vi "Integrate1D.vi"(9 "Avg N":i32, 11 "Array In":dbl[](array[numeric])) -> (3 "Array Out":dbl[](array[numeric]))   [LabVIEW 2013]
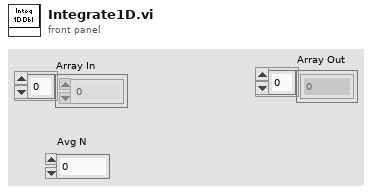
[diagram p1: front panel]
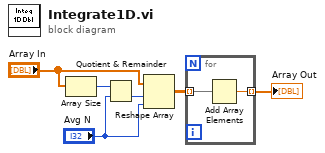
[diagram p0: block diagram]
diagram:
  n1 = Array Size(array="Array In") -> (size(s)=w2:i32)
  n2 = Quotient & Remainder(x=w2, y="Avg N") -> (floor(x/y)=w3:i32)  [unwired: 1 out]
  n3 = Reshape Array("Array In", w3, "Avg N") -> (w4:dbl[][])
  n4 = for {
    tunnel: w4 -> [w8] mode=indexing
    tunnel: [w7] -> w1 mode=indexing
    n5 = Add Array Elements(numeric array=w8) -> (sum=w7:dbl)
  }
  "Array Out" <- w1
